vi "Read Shared Variable.vi"(8 "Error In":errorcluster, 9 "Type code":i32, 10 "Refnum":refnum<k21>, 11 "Waveform in":waveform(dbl)) -> (0 "Error Out":errorcluster, 1 "status":bool, 2 "size(s)":i32[](array[numeric]), 3 "Waveform out":waveform(dbl))   [LabVIEW 2014]
doc: "<B>Copyright</B>: (c) MHWirth 2015. All rights are reserved.\n\nThis SubVI reads the shared variable and places it into Y element of the input waveform. \n\n<B>Note 1</B>: Waveform type is double. Therefore, whatever type that shared variable is, it is converted to double.\n\n<B>Note 2</B>: It does not support 1D and 2D arrays of <B>strings</B>.\n\n<B>Note 3</B>: 2D arrays are converted to 1D arrays.\n\nSupported shared variable types:\nCode 1. Boolean\nCode 2 to 5. Int8/16/32/64\nCode 6 to 9. UInt8/16/32/64\nCode 10. Double\nCode 11. Single-precision\nCode 12. String\nCode 13-23 - 1D array of above types except string\n\n<B>Error 7001</B>: Unknown Data Type - Type Code Array (Int32) contains -1 indicating an unknown data type."
uses:
  Convert 2D to 1D Boolean.vi
  Convert 2D to 1D Double.vi
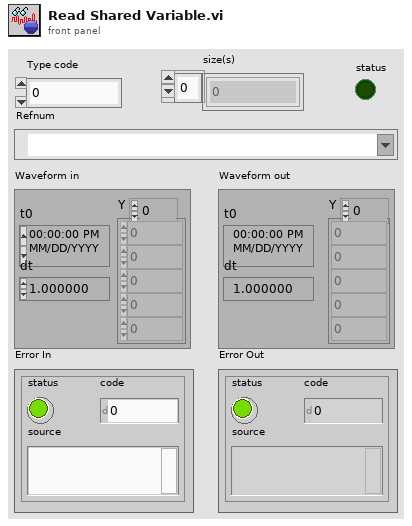
[diagram p1: front panel]
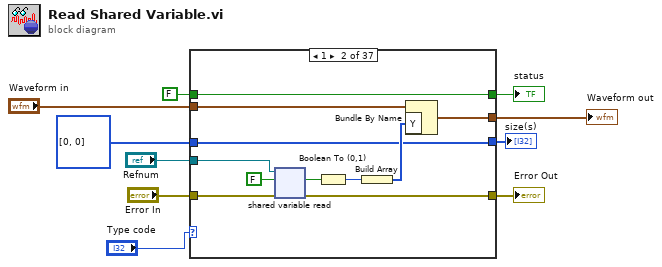
[diagram p0: block diagram]
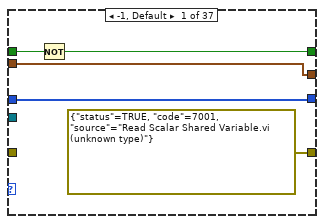
[diagram p2: hidden frame]
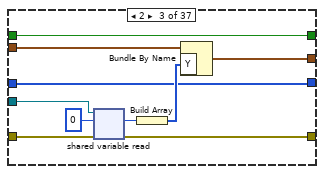
[diagram p3: hidden frame]
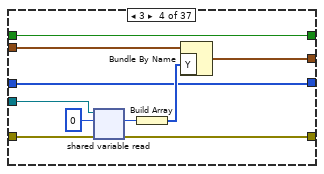
[diagram p4: hidden frame]
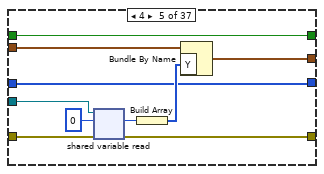
[diagram p5: hidden frame]
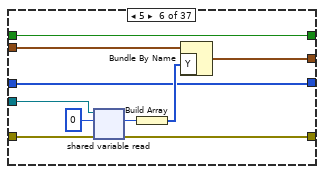
[diagram p6: hidden frame]
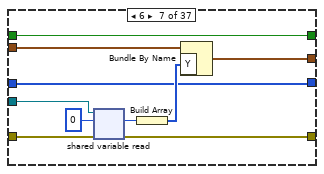
[diagram p7: hidden frame]
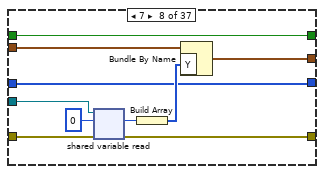
[diagram p8: hidden frame]
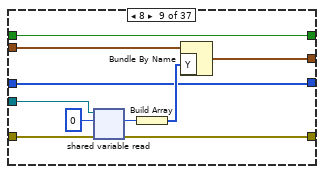
[diagram p9: hidden frame]
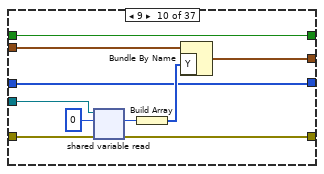
[diagram p10: hidden frame]
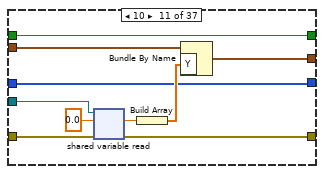
[diagram p11: hidden frame]
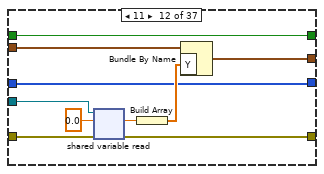
[diagram p12: hidden frame]
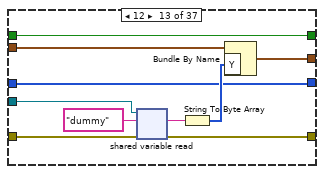
[diagram p13: hidden frame]
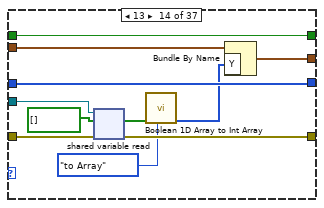
[diagram p14: hidden frame]
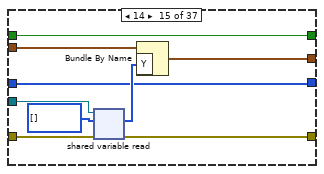
[diagram p15: hidden frame]
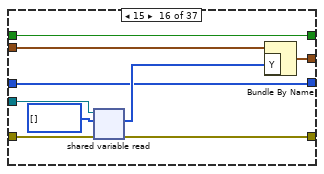
[diagram p16: hidden frame]
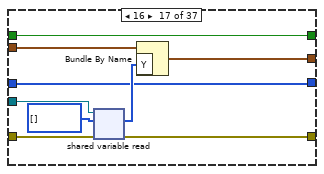
[diagram p17: hidden frame]
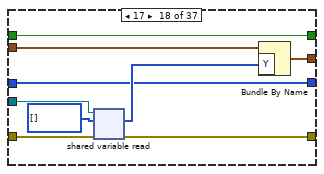
[diagram p18: hidden frame]
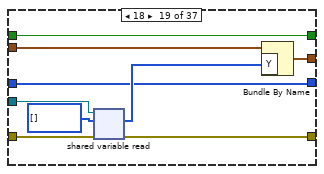
[diagram p19: hidden frame]
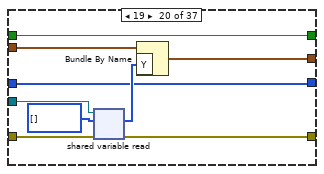
[diagram p20: hidden frame]
diagram:
  n1 = case shown="1" "Type code" {
    tunnel: [errorcluster {"status"=TRUE, "code"=7001, "source"="Read Scalar Shared Variable.vi (unknown type)"} ("error constant") w25 w35 w45 w55 w65 w75 w85 w95 w105 w115 w125 w136 w147 w156 w165 w174 w183 w192 w201 w210 w219 w228 w237 errorcluster {"status"=FALSE, "code"=7002, "source"="Read Shared Variable.vi (1D array of string not supported)"} ("Error In") w253 w263 w273 w283 w293 w303 w313 w323 w333 w343 w353 errorcluster {"status"=FALSE, "code"=7003, "source"="Read Shared Variable.vi (2D array of string not supported)"} ("Error In")] -> w9
    tunnel: [w15 w19 w30 w40 w50 w60 w70 w79 w90 w100 w110 w120 w130 w144 w153 w162 w171 w180 w189 w198 w207 w216 w225 w234 w241 w250 w260 w270 w280 w290 w300 w310 w320 w330 w340 w350 w357] -> w3
    tunnel: "Refnum" -> [_ w24 w33 w41 w51 w61 w71 w81 w91 w101 w111 w121 w134 w145 w154 w163 w172 w181 w190 w199 w208 w217 w226 w235 _ w251 w261 w271 w281 w291 w301 w311 w321 w331 w341 w351 _]
    tunnel: "Error In" -> [_ w23 w34 w42 w52 w62 w72 w82 w92 w102 w112 w122 w135 w146 w155 w164 w173 w182 w191 w200 w209 w218 w227 w236 _ w252 w262 w272 w282 w292 w302 w312 w322 w332 w342 w352 _]
    tunnel: [w12 w17 w29 w39 w48 w59 w69 w78 w89 w98 w109 w119 w129 w143 w152 w161 w170 w179 w188 w197 w206 w215 w224 w233 w240 w249 w259 w269 w279 w289 w299 w309 w319 w329 w339 w349 w356] -> w4
    tunnel: "Waveform in" -> [w12 w18 w28 w38 w49 w58 w68 w80 w88 w99 w108 w118 w128 w142 w151 w160 w169 w178 w187 w196 w205 w214 w223 w232 w240 w248 w258 w268 w278 w288 w298 w308 w318 w328 w338 w348 w356]
    tunnel: FALSE -> [w13 w19 w30 w40 w50 w60 w70 w79 w90 w100 w110 w120 w130 w144 w153 w162 w171 w180 w189 w198 w207 w216 w225 w234 w241 w250 w260 w270 w280 w290 w300 w310 w320 w330 w340 w350 w357]
    tunnel: [w11 w16 w27 w37 w47 w57 w67 w77 w87 w97 w107 w117 w127 w140 w148 w157 w166 w175 w184 w193 w202 w211 w220 w229 w238 w245 w256 w266 w275 w285 w294 w304 w314 w324 w335 w345 w354] -> w1
    tunnel: i32[] [0, 0] ("size(s)") -> [w11 w16 w27 w37 w47 w57 w67 w77 w87 w97 w107 w117 w127 w140 w148 w157 w166 w175 w184 w193 w202 w211 w220 w229 w238 _ _ _ _ _ _ _ _ _ _ _ w354]
    frame -1, Default {
      n2 = Not(x=w13) -> (.not. x?=w15:bool)
    }
    frame 1 {
      n3 = shared-variable-read(w24, w23, FALSE) -> (w25:errorcluster, w22:bool)  [unwired: 2 out]
      n4 = Boolean To (0,1)(Boolean=w22) -> (0, 1=w21:i16)
      n5 = Build Array(w21) -> (w20:i16[])
      n6 = Bundle By Name(cluster=w18, "Y"=w20) -> (w17:waveform(dbl))
    }
    frame 2 {
      n7 = shared-variable-read(w33, w34, i8 0) -> (w35:errorcluster, w32:i8)  [unwired: 2 out]
      n8 = Build Array(w32) -> (w31:i8[])
      n9 = Bundle By Name(cluster=w28, "Y"=w31) -> (w29:waveform(dbl))
    }
    frame 3 {
      n10 = shared-variable-read(w41, w42, i16 0) -> (w45:errorcluster, w44:i16)  [unwired: 2 out]
      n11 = Build Array(w44) -> (w43:i16[])
      n12 = Bundle By Name(cluster=w38, "Y"=w43) -> (w39:waveform(dbl))
    }
    frame 4 {
      n13 = shared-variable-read(w51, w52, 0) -> (w55:errorcluster, w54:i32)  [unwired: 2 out]
      n14 = Build Array(w54) -> (w53:i32[])
      n15 = Bundle By Name(cluster=w49, "Y"=w53) -> (w48:waveform(dbl))
    }
    frame 5 {
      n16 = shared-variable-read(w61, w62, i64 0) -> (w65:errorcluster, w64:i64)  [unwired: 2 out]
      n17 = Build Array(w64) -> (w63:i64[])
      n18 = Bundle By Name(cluster=w58, "Y"=w63) -> (w59:waveform(dbl))
    }
    frame 6 {
      n19 = shared-variable-read(w71, w72, u8 0) -> (w75:errorcluster, w74:u8)  [unwired: 2 out]
      n20 = Build Array(w74) -> (w73:u8[])
      n21 = Bundle By Name(cluster=w68, "Y"=w73) -> (w69:waveform(dbl))
    }
    frame 7 {
      n22 = shared-variable-read(w81, w82, u16 0) -> (w85:errorcluster, w84:u16)  [unwired: 2 out]
      n23 = Build Array(w84) -> (w83:u16[])
      n24 = Bundle By Name(cluster=w80, "Y"=w83) -> (w78:waveform(dbl))
    }
    frame 8 {
      n25 = shared-variable-read(w91, w92, u32 0) -> (w95:errorcluster, w94:u32)  [unwired: 2 out]
      n26 = Build Array(w94) -> (w93:u32[])
      n27 = Bundle By Name(cluster=w88, "Y"=w93) -> (w89:waveform(dbl))
    }
    frame 9 {
      n28 = shared-variable-read(w101, w102, u64 0) -> (w105:errorcluster, w104:u64)  [unwired: 2 out]
      n29 = Build Array(w104) -> (w103:u64[])
      n30 = Bundle By Name(cluster=w99, "Y"=w103) -> (w98:waveform(dbl))
    }
    frame 10 {
      n31 = shared-variable-read(w111, w112, 0.0) -> (w115:errorcluster, w114:dbl)  [unwired: 2 out]
      n32 = Build Array(w114) -> (w113:dbl[])
      n33 = Bundle By Name(cluster=w108, "Y"=w113) -> (w109:waveform(dbl))
    }
    frame 11 {
      n34 = shared-variable-read(w121, w122, sgl 0.0) -> (w125:errorcluster, w124:sgl)  [unwired: 2 out]
      n35 = Build Array(w124) -> (w123:sgl[])
      n36 = Bundle By Name(cluster=w118, "Y"=w123) -> (w119:waveform(dbl))
    }
    frame 12 {
      n37 = shared-variable-read(w134, w135, "dummy") -> (w136:errorcluster, w132:string)  [unwired: 2 out]
      n38 = String To Byte Array(string=w132) -> (unsigned byte array=w131:u8[])
      n39 = Bundle By Name(cluster=w128, "Y"=w131) -> (w129:waveform(dbl))
    }
    frame 13 {
      n40 = shared-variable-read(w145, w146, bool[] []) -> (w147:errorcluster, w139:bool[])  [unwired: 2 out]
      n41 = call "Boolean 1D Array to Int Array.vi"("Mode"=enum16{"to Array", "to Number"}."to Array" ("Enum"), "Array of Boolean"=w139) -> ("Array out"=w137:u32[])  [unwired: 8 in]
      n42 = Bundle By Name(cluster=w142, "Y"=w137) -> (w143:waveform(dbl))
    }
    frame 14 {
      n43 = shared-variable-read(w154, w155, i8[] []) -> (w156:errorcluster, w149:i8[])  [unwired: 2 out]
      n44 = Bundle By Name(cluster=w151, "Y"=w149) -> (w152:waveform(dbl))
    }
    frame 15 {
      n45 = shared-variable-read(w163, w164, i16[] []) -> (w165:errorcluster, w158:i16[])  [unwired: 2 out]
      n46 = Bundle By Name(cluster=w160, "Y"=w158) -> (w161:waveform(dbl))
    }
    frame 16 {
      n47 = shared-variable-read(w172, w173, i32[] []) -> (w174:errorcluster, w167:i32[])  [unwired: 2 out]
      n48 = Bundle By Name(cluster=w169, "Y"=w167) -> (w170:waveform(dbl))
    }
    frame 17 {
      n49 = shared-variable-read(w181, w182, i64[] []) -> (w183:errorcluster, w176:i64[])  [unwired: 2 out]
      n50 = Bundle By Name(cluster=w178, "Y"=w176) -> (w179:waveform(dbl))
    }
    frame 18 {
      n51 = shared-variable-read(w190, w191, u8[] []) -> (w192:errorcluster, w185:u8[])  [unwired: 2 out]
      n52 = Bundle By Name(cluster=w187, "Y"=w185) -> (w188:waveform(dbl))
    }
    frame 19 {
      n53 = shared-variable-read(w199, w200, u16[] []) -> (w201:errorcluster, w194:u16[])  [unwired: 2 out]
      n54 = Bundle By Name(cluster=w196, "Y"=w194) -> (w197:waveform(dbl))
    }
    frame 20 {
      n55 = shared-variable-read(w208, w209, u32[] []) -> (w210:errorcluster, w203:u32[])  [unwired: 2 out]
      n56 = Bundle By Name(cluster=w205, "Y"=w203) -> (w206:waveform(dbl))
    }
    frame 21 {
      n57 = shared-variable-read(w217, w218, u64[] []) -> (w219:errorcluster, w212:u64[])  [unwired: 2 out]
      n58 = Bundle By Name(cluster=w214, "Y"=w212) -> (w215:waveform(dbl))
    }
    frame 22 {
      n59 = shared-variable-read(w226, w227, dbl[] []) -> (w228:errorcluster, w221:dbl[])  [unwired: 2 out]
      n60 = Bundle By Name(cluster=w223, "Y"=w221) -> (w224:waveform(dbl))
    }
    frame 23 {
      n61 = shared-variable-read(w235, w236, sgl[] []) -> (w237:errorcluster, w230:sgl[])  [unwired: 2 out]
      n62 = Bundle By Name(cluster=w232, "Y"=w230) -> (w233:waveform(dbl))
    }
    frame 24 {
    }
    frame 25 {
      n63 = shared-variable-read(w251, w252, bool[][] []) -> (w253:errorcluster, w246:bool[][])  [unwired: 2 out]
      n64 = call-poly "Convert 2D to 1D.vi"("2D Array"=w246) -> ("size(s)"=w245:i32[], "1D Array"=w244:bool[])  [unwired: 9 in]
      n65 = call "Boolean 1D Array to Int Array.vi"("Mode"=enum16{"to Array", "to Number"}."to Array" ("Enum"), "Array of Boolean"=w244) -> ("Array out"=w242:u32[])  [unwired: 8 in]
      n66 = Bundle By Name(cluster=w248, "Y"=w242) -> (w249:waveform(dbl))
    }
    frame 26 {
      n67 = shared-variable-read(w261, w262, i8[][] []) -> (w263:errorcluster, w254:i8[][])  [unwired: 2 out]
      n68 = call-poly "Convert 2D to 1D.vi"("2D Array"=w254) -> ("size(s)"=w256:i32[], "1D Array"=w255:dbl[])  [unwired: 9 in]
      n69 = Bundle By Name(cluster=w258, "Y"=w255) -> (w259:waveform(dbl))
    }
    frame 27 {
      n70 = shared-variable-read(w271, w272, i16[][] []) -> (w273:errorcluster, w264:i16[][])  [unwired: 2 out]
      n71 = call-poly "Convert 2D to 1D.vi"("2D Array"=w264) -> ("size(s)"=w266:i32[], "1D Array"=w265:dbl[])  [unwired: 9 in]
      n72 = Bundle By Name(cluster=w268, "Y"=w265) -> (w269:waveform(dbl))
    }
    frame 28 {
      n73 = shared-variable-read(w281, w282, i32[][] []) -> (w283:errorcluster, w274:i32[][])  [unwired: 2 out]
      n74 = call-poly "Convert 2D to 1D.vi"("2D Array"=w274) -> ("size(s)"=w275:i32[], "1D Array"=w276:dbl[])  [unwired: 9 in]
      n75 = Bundle By Name(cluster=w278, "Y"=w276) -> (w279:waveform(dbl))
    }
    frame 29 {
      n76 = shared-variable-read(w291, w292, i64[][] []) -> (w293:errorcluster, w284:i64[][])  [unwired: 2 out]
      n77 = call-poly "Convert 2D to 1D.vi"("2D Array"=w284) -> ("size(s)"=w285:i32[], "1D Array"=w286:dbl[])  [unwired: 9 in]
      n78 = Bundle By Name(cluster=w288, "Y"=w286) -> (w289:waveform(dbl))
    }
    frame 30 {
      n79 = shared-variable-read(w301, w302, u8[][] []) -> (w303:errorcluster, w295:u8[][])  [unwired: 2 out]
      n80 = call-poly "Convert 2D to 1D.vi"("2D Array"=w295) -> ("size(s)"=w294:i32[], "1D Array"=w296:dbl[])  [unwired: 9 in]
      n81 = Bundle By Name(cluster=w298, "Y"=w296) -> (w299:waveform(dbl))
    }
    frame 31 {
      n82 = shared-variable-read(w311, w312, u16[][] []) -> (w313:errorcluster, w305:u16[][])  [unwired: 2 out]
      n83 = call-poly "Convert 2D to 1D.vi"("2D Array"=w305) -> ("size(s)"=w304:i32[], "1D Array"=w306:dbl[])  [unwired: 9 in]
      n84 = Bundle By Name(cluster=w308, "Y"=w306) -> (w309:waveform(dbl))
    }
    frame 32 {
      n85 = shared-variable-read(w321, w322, u32[][] []) -> (w323:errorcluster, w315:u32[][])  [unwired: 2 out]
      n86 = call-poly "Convert 2D to 1D.vi"("2D Array"=w315) -> ("size(s)"=w314:i32[], "1D Array"=w316:dbl[])  [unwired: 9 in]
      n87 = Bundle By Name(cluster=w318, "Y"=w316) -> (w319:waveform(dbl))
    }
    frame 33 {
      n88 = shared-variable-read(w331, w332, u64[][] []) -> (w333:errorcluster, w325:u64[][])  [unwired: 2 out]
      n89 = call-poly "Convert 2D to 1D.vi"("2D Array"=w325) -> ("size(s)"=w324:i32[], "1D Array"=w326:dbl[])  [unwired: 9 in]
      n90 = Bundle By Name(cluster=w328, "Y"=w326) -> (w329:waveform(dbl))
    }
    frame 34 {
      n91 = shared-variable-read(w341, w342, dbl[][] []) -> (w343:errorcluster, w334:dbl[][])  [unwired: 2 out]
      n92 = call-poly "Convert 2D to 1D.vi"("2D Array"=w334) -> ("size(s)"=w335:i32[], "1D Array"=w336:dbl[])  [unwired: 9 in]
      n93 = Bundle By Name(cluster=w338, "Y"=w336) -> (w339:waveform(dbl))
    }
    frame 35 {
      n94 = shared-variable-read(w351, w352, sgl[][] []) -> (w353:errorcluster, w344:sgl[][])  [unwired: 2 out]
      n95 = call-poly "Convert 2D to 1D.vi"("2D Array"=w344) -> ("size(s)"=w345:i32[], "1D Array"=w346:dbl[])  [unwired: 9 in]
      n96 = Bundle By Name(cluster=w348, "Y"=w346) -> (w349:waveform(dbl))
    }
    frame 36 {
    }
  }
  "Error Out" <- w9
  "Waveform out" <- w4
  "status" <- w3
  "size(s)" <- w1
